vi "12.4 MorphReconstruct-Binary.vi"() -> ()   [LabVIEW 2016]
doc: "This example shows how to use the Edge Tool in NI Vision. The Edge Tool finds edges (or sharp transitions in the pixels values) along a given line or ROI profile. The Edge Tool is a precursor function to many of the gauging and inspection tasks. For example, the location of the edges found along a line profile across an object can interpreted as the boundaries of the object whose dimensions have to be measured for a gauging application or the presence of a crack in the surface of an object for an inspection application."
uses:
  <vilib>/vision/NI_Vision_Development_Module.lvlib
panel:
  in  "Operation":enum32{"Dilate", "Erode"}(ring)
  in  "Tab":T1(tab)
  out "Src":T2(plugin-control)
  out "Bin":T2(plugin-control)
  out "Map":T2(plugin-control)
  out "Marker":T2(plugin-control)
  out "Dst":T2(plugin-control)
  in  "Marker Thicker":cluster{"Lower value":sgl, "Upper value":sgl}={"Lower value"=46.0, "Upper value"=200.0}
  in  "Connectivity":bool=TRUE
  in  "Stop":bool
  # "Instruction:\nRun program, check the image created in each steps.\n\nNote the reconstruction can only work correctly when operation is be Dilate for this case;\n\nChange the marker Thicker to check out the different Marker image generated."
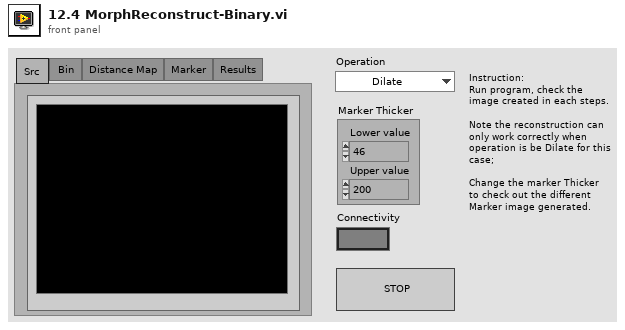
[diagram p1: front panel]
types:
  T1 = enum32{"Src ", "Bin ", "Distance Map", "Marker", "Results"}
  T2 = typedef "IMAQ Image.ctl" = refnum<image>
  T3 = cluster{"Operation":enum32{"Dilate", "Erode"}, "Marker Thicker":cluster{"Lower value":sgl, "Upper value":sgl}, "Connectivity":bool}
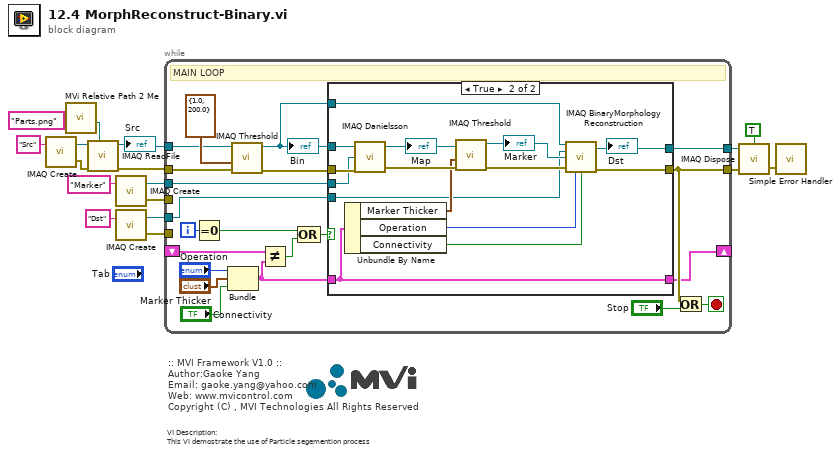
[diagram p0: block diagram]
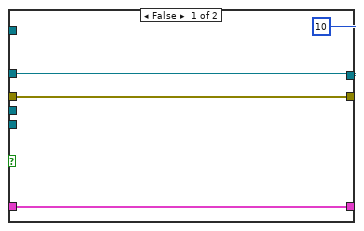
[diagram p2: hidden frame]
diagram:
  # "VI Description:\nThis VI demostrate the use of Particle segemention process"
  # ":: MVI Framework V1.0 ::\nAuthor:Gaoke Yang\nEmail: gaoke.yang@yahoo.com\nWeb: www.mvicontrol.com\nCopyright (C) , MVI Technologies All Rights Reserved"
  n1 = call "IMAQ Create"("Image Name"="Src") -> ("New Image"=w16:T2, "error out"=w15:errorcluster)  [unwired: 4 in]
  n2 = call "MVi Relative Path 2 Me.vi"("Relative Path"="Parts.png" ("name or relative path")) -> ("Appended Dir"=w11:path)  [unwired: 5 in, 1 out]
  n3 = call "IMAQ ReadFile"("File Path"=w11, "error in (no error)"=w15, "Image"=w16) -> ("error out"=w5:errorcluster, "Image Out"=w4:T2)  [unwired: 4 in, 3 out]
  "Src" <- w4
  n4 = call "IMAQ Create"("Image Name"="Marker") -> ("New Image"=w8:T2, "error out"=w7:errorcluster)  [unwired: 4 in]
  n5 = call "IMAQ Create"("Image Name"="Dst") -> ("New Image"=w2:T2, "error out"=w1:errorcluster)  [unwired: 4 in]
  n6 = while "MAIN LOOP" {
    tunnel: w4 -> [w21]
    tunnel: w5 -> [w24]
    tunnel: [w35] -> w14
    tunnel: [w36] -> w13
    shift-right: [w32] -> _
    shift-left: _ -> [w30]
    tunnel: w8 -> [w20]
    tunnel: w7 -> [_]
    tunnel: w2 -> [w25]
    tunnel: w1 -> [_]
    i -> [w34]
    stop <- w37 stop-if-true
    # "MAIN LOOP"
    n7 = Equal To 0?(x=w34) -> (x = 0?=w31:bool)
    n8 = Bundle("Operation"="Operation", "Marker Thicker"="Marker Thicker", "Connectivity"="Connectivity") -> (w28:T3)  [unwired: 1 in]
    n9 = call "IMAQ Threshold"("error in (no error)"=w24, "Range"=cluster{"Lower value":sgl, "Upper value":sgl} {"Lower value"=1.0, "Upper value"=200.0}, "Image Src"=w21) -> ("error out"=w22:errorcluster, "Image Dst Out"=w19:T2)  [unwired: 7 in]
    "Bin" <- w19
    n10 = Not Equal?(x=w30, y=w28) -> (x != y?=w29:bool)
    n11 = Compound Arithmetic op=OR(w31, w29) -> (w33:bool)
    n12 = case shown="True" w33 {
      tunnel: w22 -> [w41 w54]
      tunnel: w19 -> [w42 w53]
      tunnel: [w42 w46] -> w36
      tunnel: [w41 w47] -> w35
      tunnel: [w39 w57] -> w32
      tunnel: w28 -> [w39 w57]
      tunnel: w25 -> [_ w48]
      tunnel: w19 -> [_ w49]
      tunnel: w20 -> [_ w45]
      frame False {
        n13 = Wait (ms)(milliseconds to wait=u32 10) -> ()  [unwired: 1 out]
      }
      frame True {
        n14 = Unbundle By Name(w57) -> ("Marker Thicker"=w52:cluster{"Lower value":sgl, "Upper value":sgl}, "Operation"=w44:enum32{"Dilate", "Erode"}, "Connectivity"=w43:bool)
        n15 = call "IMAQ Danielsson"("error in (no error)"=w54, "Image Dst"=w45, "Image Src"=w53) -> ("error out"=w56:errorcluster, "Image Dst Out"=w51:T2)  [unwired: 1 in]
        "Map" <- w51
        n16 = call "IMAQ Threshold"("error in (no error)"=w56, "Range"=w52, "Image Src"=w51) -> ("error out"=w55:errorcluster, "Image Dst Out"=w50:T2)  [unwired: 3 in, 4 out]
        "Marker" <- w50
        n17 = call "IMAQ BinaryMorphology Reconstruction"("Image Src"=w49, "Image Dst"=w48, "Image Marker"=w50, "error in (no error)"=w55, "Operation"=w44, "Connectivity 4/8 (8)"=w43) -> ("Image Dst Out"=w46:T2, "error out"=w47:errorcluster)  [unwired: 8 in]
        "Dst" <- w46
      }
    }
    n18 = Or(x=w35, y="Stop") -> (x .or. y?=w37:bool)
  }
  n19 = call "IMAQ Dispose"("All Images? (No)"=TRUE, "Image"=w13, "error in (no error)"=w14) -> ("error out"=w10:errorcluster)  [unwired: 3 in]
  n20 = call <vilib>:"Simple Error Handler.vi"("error in (no error)"=w10) -> ()  [unwired: 4 in, 5 out]
